vi "Open Swerve Drive.vi"() -> ()   [LabVIEW 2016, in "CAN Talon SRX Swerve.lvlib"]
uses:
  CAN Talon SRX Swerve.lvlib
  <vilib>/Rock Robotics/WPI/Encoder/WPI_EncoderType.ctl
  <vilib>/Rock Robotics/WPI/ThirdParty/CanMotor/TalonSRX/WPI_CANTalonSRX_APIControlMode.ctl
  <vilib>/Rock Robotics/SystemInterfaces/AI/FPGA_AIChannel.ctl
  <vilib>/Rock Robotics/WPI/Counter/WPI_CounterDigitalInputToDigitalSource.vi
  <vilib>/Rock Robotics/SystemInterfaces/DIO/FPGA_DIOChannel.ctl
panel:
  in  "Invert Direction 2":bool
  in  "Decoding Type 2":T1=enum."4x"
  in  "DistancePerCount 2":dbl=0.0023
  in  "Invert Direction":bool
  in  "Decoding Type":T1=enum."4x"
  in  "DistancePerCount":dbl=0.0023
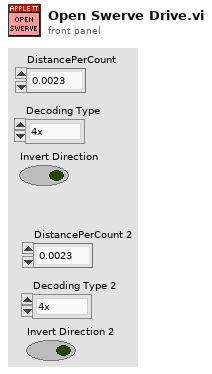
[diagram p1: front panel]
types:
  T1 = typedef "WPI_EncoderType.ctl" = enum16{"1x", "2x", "4x"}
  T2 = typedef "WPI_CANTalonSRX_APIControlMode.ctl" = enum8{"Percent VBus", "Speed", "Position", "Slave", "Unchanged / Invalid", "Voltage Compensation", "Current", "Motion Profile", "Motion Magic"}
  T3 = typedef "WPI_MotorControlDeviceRef.ctl" = cluster{"DeviceStatus":errorcluster, "Type":T4, "PWM":cluster{"PWM Channel":T5, "DeadBand":T6}, "CAN":cluster{"Device Number":u8, "SetOutput VI Ref":variant, "GetOutput VI Ref":variant, "Enable VI Ref":variant, "Disable VI Ref":variant, "Data":variant}, "Invert":bool}
  T4 = typedef "WPI_MotorControlType.ctl" = enum16{"PWM", "CAN"}
  T5 = typedef "FPGA_DIOPWMChannel.ctl" = enum8{"PWM 0", "PWM 1", "PWM 2", "PWM 3", "PWM 4", "PWM 5", "PWM 6", "PWM 7", "PWM 8", "PWM 9", "PWM MXP 0", "PWM MXP 1", "PWM MXP 2", "PWM MXP 3", "PWM MXP 4", "PWM MXP 5", "PWM MXP 6", "PWM MXP 7", "PWM MXP 8", "PWM MXP 9", "Invalid"}
  T6 = typedef "WPI_PWMDeadband.ctl" = cluster{"Name":string, "maxPositivePwm":i32, "minPositivePwm":i32, "centerPwm":i32, "maxNegativePwm":i32, "minNegativePwm":i32, "angularRange":u16}
  T7 = typedef "FPGA_DIOChannel.ctl" = enum8{"DIO 0", "DIO 1", "DIO 2", "DIO 3", "DIO 4", "DIO 5", "DIO 6", "DIO 7", "DIO 8", "DIO 9", "DIO MXP 0", "DIO MXP 1", "DIO MXP 2", "DIO MXP 3", "DIO MXP 4", "DIO MXP 5", "DIO MXP 6", "DIO MXP 7", "DIO MXP 8", "DIO MXP 9", "DIO MXP 10", "DIO MXP 11", "DIO MXP 12", "DIO MXP 13", "DIO MXP 14", "DIO MXP 15", "SPI Port CS1", "SPI Port CS2", "SPI Port CS3", "SPI Port MISO", "SPI Port MOSI", "Invalid"}
  T8 = typedef "FPGA_AIChannel.ctl" = enum8{"AI 0", "AI 1", "AI 2", "AI 3", "AI MXP 0", "AI MXP 1", "AI MXP 2", "AI MXP 3", "Invalid"}
  T9 = typedef "WPI_AnalogChannelDevRef.ctl" = cluster{"DevStatus":errorcluster, "Analog Channel":T8}
  T10 = typedef "WPI_DigitalInputDevRef.ctl" = cluster{"DevStatus":errorcluster, "DIO Channel":T7}
  T11 = typedef "FPGA_CounterEncoderSourceConvertionLVSourceType.ctl" = cluster{"DevStatus":errorcluster, "AnalogTriggerMode?":bool, "DigitalMode":cluster{"DIO Channel":T12}, "AnalogTriggerMode":cluster{"AnalogTriggerIndex":T13, "OutputType":T14}}
  T12 = typedef "FPGA_DIODigitalSourceChannel.ctl" = enum8{"DIO 0", "DIO 1", "DIO 2", "DIO 3", "DIO 4", "DIO 5", "DIO 6", "DIO 7", "DIO 8", "DIO 9", "DIO MXP 0", "DIO MXP 1", "DIO MXP 2", "DIO MXP 3", "DIO MXP 4", "DIO MXP 5", "DIO MXP 6", "DIO MXP 7", "DIO MXP 8", "DIO MXP 9", "DIO MXP 10", "DIO MXP 11", "DIO MXP 12", "DIO MXP 13", "DIO MXP 14", "DIO MXP 15", "Disabled"}
  T13 = typedef "FPGA_AnalogTriggerIndex.ctl" = enum8{"Trig 0", "Trig 1", "Trig 2", "Trig 3", "Trig 4", "Trig 5", "Trig 6", "Trig 7", "Invalid"}
  T14 = typedef "FPGA_AnalogTriggerOutType.ctl" = enum16{"InWindow", "TriggerState", "Rising", "Falling"}
  T15 = typedef "WPI_EncoderDevRef.ctl" = cluster{"DevStatus":errorcluster, "EncoderIndex":T16, "CounterIndex":T17, "DistancePerCount":dbl, "Decoding Type":T1}
  T16 = typedef "FPGA_EncoderIdx.ctl" = enum8{"Enc 0", "Enc 1", "Enc 2", "Enc 3", "Enc 4", "Enc 5", "Enc 6", "Enc 7", "Invalid"}
  T17 = typedef "FPGA_CounterCtrSystemIndex.ctl" = enum8{"Ctr 0", "Ctr 1", "Ctr 2", "Ctr 3", "Ctr 4", "Ctr 5", "Ctr 6", "Ctr 7", "Invalid"}
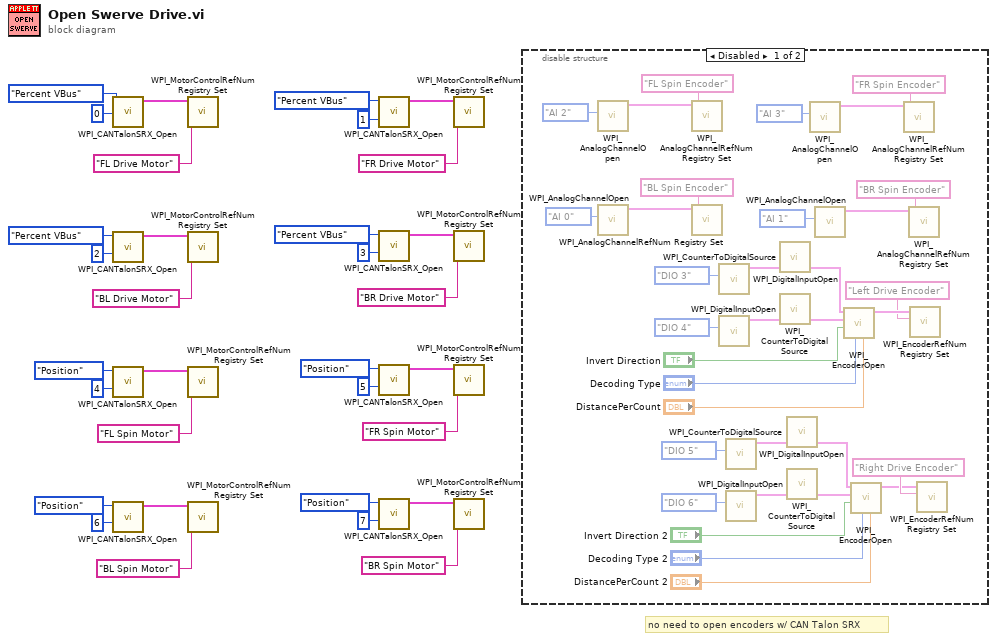
[diagram p0: block diagram]
diagram:
  # "no need to open encoders w/ CAN Talon SRX"
  n1 = call <vilib>:"WPI_CANTalonSRX_Open.vi"("Device Number"=u8 0, "Control Mode"=WPI_CANTalonSRX_APIControlMode."Percent VBus") -> ("CAN Talon SRX Ref"=w32:T3)  [unwired: 8 in, 1 out]
  n2 = call <vilib>:"WPI_CANTalonSRX_Open.vi"("Device Number"=u8 2, "Control Mode"=WPI_CANTalonSRX_APIControlMode."Percent VBus") -> ("CAN Talon SRX Ref"=w31:T3)  [unwired: 8 in, 1 out]
  n3 = call <vilib>:"WPI_CANTalonSRX_Open.vi"("Device Number"=u8 4, "Control Mode"=WPI_CANTalonSRX_APIControlMode."Position") -> ("CAN Talon SRX Ref"=w30:T3)  [unwired: 8 in, 1 out]
  n4 = call <vilib>:"WPI_CANTalonSRX_Open.vi"("Device Number"=u8 6, "Control Mode"=WPI_CANTalonSRX_APIControlMode."Position") -> ("CAN Talon SRX Ref"=w29:T3)  [unwired: 8 in, 1 out]
  n5 = call <vilib>:"WPI_MotorControlRefNum Registry Set.vi"("refnum name"="FL Drive Motor", "MotorControlDevRef"=w32) -> ()  [unwired: 8 in, 2 out]
  n6 = call <vilib>:"WPI_MotorControlRefNum Registry Set.vi"("refnum name"="BL Drive Motor", "MotorControlDevRef"=w31) -> ()  [unwired: 8 in, 2 out]
  n7 = call <vilib>:"WPI_MotorControlRefNum Registry Set.vi"("refnum name"="FL Spin Motor", "MotorControlDevRef"=w30) -> ()  [unwired: 8 in, 2 out]
  n8 = call <vilib>:"WPI_MotorControlRefNum Registry Set.vi"("refnum name"="BL Spin Motor", "MotorControlDevRef"=w29) -> ()  [unwired: 8 in, 2 out]
  n9 = call <vilib>:"WPI_CANTalonSRX_Open.vi"("Device Number"=u8 1, "Control Mode"=WPI_CANTalonSRX_APIControlMode."Percent VBus") -> ("CAN Talon SRX Ref"=w28:T3)  [unwired: 8 in, 1 out]
  n10 = call <vilib>:"WPI_CANTalonSRX_Open.vi"("Device Number"=u8 3, "Control Mode"=WPI_CANTalonSRX_APIControlMode."Percent VBus") -> ("CAN Talon SRX Ref"=w27:T3)  [unwired: 8 in, 1 out]
  n11 = call <vilib>:"WPI_CANTalonSRX_Open.vi"("Device Number"=u8 5, "Control Mode"=WPI_CANTalonSRX_APIControlMode."Position") -> ("CAN Talon SRX Ref"=w26:T3)  [unwired: 8 in, 1 out]
  n12 = call <vilib>:"WPI_CANTalonSRX_Open.vi"("Device Number"=u8 7, "Control Mode"=WPI_CANTalonSRX_APIControlMode."Position") -> ("CAN Talon SRX Ref"=w25:T3)  [unwired: 8 in, 1 out]
  n13 = call <vilib>:"WPI_MotorControlRefNum Registry Set.vi"("refnum name"="FR Drive Motor", "MotorControlDevRef"=w28) -> ()  [unwired: 8 in, 2 out]
  n14 = call <vilib>:"WPI_MotorControlRefNum Registry Set.vi"("refnum name"="BR Drive Motor", "MotorControlDevRef"=w27) -> ()  [unwired: 8 in, 2 out]
  n15 = call <vilib>:"WPI_MotorControlRefNum Registry Set.vi"("refnum name"="FR Spin Motor", "MotorControlDevRef"=w26) -> ()  [unwired: 8 in, 2 out]
  n16 = call <vilib>:"WPI_MotorControlRefNum Registry Set.vi"("refnum name"="BR Spin Motor", "MotorControlDevRef"=w25) -> ()  [unwired: 8 in, 2 out]
  n17 = disable-structure shown="Disabled" {
    frame Disabled {
      n18 = call <vilib>:"WPI_AnalogChannelOpen.vi"("Analog Channel"=FPGA_AIChannel."AI 2") -> ("AIDeviceRef"=w62:T9)  [unwired: 9 in, 1 out]
      n19 = call <vilib>:"WPI_AnalogChannelOpen.vi"("Analog Channel"=FPGA_AIChannel."AI 0") -> ("AIDeviceRef"=w65:T9)  [unwired: 9 in, 1 out]
      n20 = call <vilib>:"WPI_AnalogChannelRefNum Registry Set.vi"("refnum name"="FL Spin Encoder", "AIDeviceRef"=w62) -> ()  [unwired: 8 in, 2 out]
      n21 = call <vilib>:"WPI_AnalogChannelRefNum Registry Set.vi"("refnum name"="BL Spin Encoder", "AIDeviceRef"=w65) -> ()  [unwired: 8 in, 2 out]
      n22 = call <vilib>:"WPI_DigitalInputOpen.vi"("DIO Channel"=FPGA_DIOChannel."DIO 3") -> ("DigitalInputDevRef"=w52:T10)  [unwired: 1 in, 9 out]
      n23 = call <vilib>:"WPI_DigitalInputOpen.vi"("DIO Channel"=FPGA_DIOChannel."DIO 4") -> ("DigitalInputDevRef"=w53:T10)  [unwired: 1 in, 9 out]
      n24 = call <vilib>:"WPI_DigitalInputOpen.vi"("DIO Channel"=FPGA_DIOChannel."DIO 5") -> ("DigitalInputDevRef"=w35:T10)  [unwired: 1 in, 9 out]
      n25 = call <vilib>:"WPI_DigitalInputOpen.vi"("DIO Channel"=FPGA_DIOChannel."DIO 6") -> ("DigitalInputDevRef"=w34:T10)  [unwired: 1 in, 9 out]
      n26 = call-poly <vilib>:"WPI_CounterToDigitalSource.vi"("DigitalInputDevRef"=w52) -> ("Digital Source"=w51:T11)  [unwired: 6 out]
      n27 = call-poly <vilib>:"WPI_CounterToDigitalSource.vi"("DigitalInputDevRef"=w53) -> ("Digital Source"=w54:T11)  [unwired: 6 out]
      n28 = call-poly <vilib>:"WPI_CounterToDigitalSource.vi"("DigitalInputDevRef"=w35) -> ("Digital Source"=w36:T11)  [unwired: 6 out]
      n29 = call-poly <vilib>:"WPI_CounterToDigitalSource.vi"("DigitalInputDevRef"=w34) -> ("Digital Source"=w33:T11)  [unwired: 6 out]
      n30 = call <vilib>:"WPI_AnalogChannelOpen.vi"("Analog Channel"=FPGA_AIChannel."AI 3") -> ("AIDeviceRef"=w59:T9)  [unwired: 9 in, 1 out]
      n31 = call <vilib>:"WPI_AnalogChannelOpen.vi"("Analog Channel"=FPGA_AIChannel."AI 1") -> ("AIDeviceRef"=w56:T9)  [unwired: 9 in, 1 out]
      n32 = call <vilib>:"WPI_EncoderOpen.vi"("DistancePerCount"="DistancePerCount", "Decoding Type"="Decoding Type", "Invert Direction (False)"="Invert Direction", "BSource"=w54, "ASource"=w51) -> ("EncoderDevRef"=w45:T15)  [unwired: 3 in, 3 out]
      n33 = call <vilib>:"WPI_EncoderOpen.vi"("DistancePerCount"="DistancePerCount 2", "Decoding Type"="Decoding Type 2", "Invert Direction (False)"="Invert Direction 2", "BSource"=w33, "ASource"=w36) -> ("EncoderDevRef"=w42:T15)  [unwired: 3 in, 3 out]
      n34 = call <vilib>:"WPI_AnalogChannelRefNum Registry Set.vi"("refnum name"="FR Spin Encoder", "AIDeviceRef"=w59) -> ()  [unwired: 8 in, 2 out]
      n35 = call <vilib>:"WPI_AnalogChannelRefNum Registry Set.vi"("refnum name"="BR Spin Encoder", "AIDeviceRef"=w56) -> ()  [unwired: 8 in, 2 out]
      n36 = call <vilib>:"WPI_EncoderRefNum Registry Set.vi"("refnum name"="Left Drive Encoder", "EncoderDevRef"=w45) -> ()  [unwired: 8 in, 2 out]
      n37 = call <vilib>:"WPI_EncoderRefNum Registry Set.vi"("refnum name"="Right Drive Encoder", "EncoderDevRef"=w42) -> ()  [unwired: 8 in, 2 out]
    }
    frame Enabled {
    }
  }
